vi "convert param indicies to typedef data.vi"(8 "error in":errorcluster, 11 "Parameter Mapping Info":T1) -> (0 "error out":errorcluster, 3 "Parameters to process":T2)   [LabVIEW 2013, in "fixed channel tag bus module.lvclass"]
uses:
  fixed channel tag bus module.lvclass
  parameters.ctl
  Utilities/Cluster to Tag Bus Scripts/Channel Run Time Mapping Info.ctl
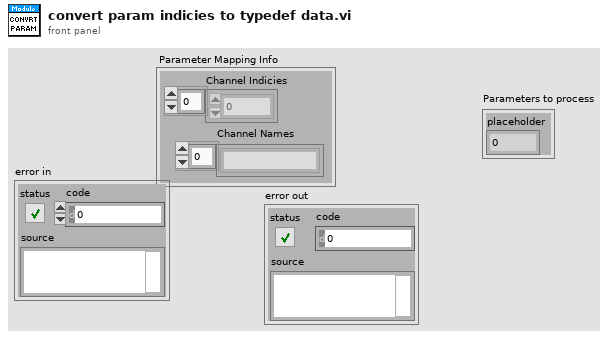
[diagram p1: front panel]
types:
  T1 = typedef "Channel Run Time Mapping Info.ctl" = cluster{"Channel Indicies":i32[], "Channel Names":string[]}
  T2 = typedef "fixed channel tag bus module.lvclass/parameters.ctl" = cluster{"placeholder":i32}
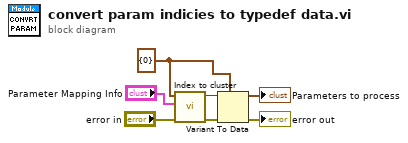
[diagram p0: block diagram]
diagram:
  w3 = T2 {"placeholder"=0} ("Parameters to process")
  n1 = call "Index to cluster.vi"("error in"="error in", "Input Mapping Info"="Parameter Mapping Info", "Variant in"=w3) -> ("error out"=w5:errorcluster, "Variant out"=w7:variant)  [unwired: 7 in]
  n2 = Variant To Data(error in=w5, type=w3, Variant=w7) -> (data=→"Parameters to process":T2, error out=→"error out":errorcluster)
